vi "Handshake.vi"(5 "error in":T1) -> (19 "error out":T1)   [LabVIEW 2016]
doc: "If the path mode is waiting for a manual handshake, this VI will give this handshake and the path will be continued."
uses:
  Controls/Error_Out.ctl
  Files_ASC500/DLL/ASC500_RemoteControlV27.dll
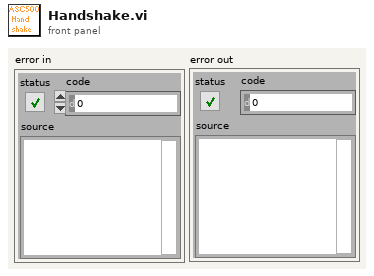
[diagram p1: front panel]
types:
  T1 = typedef "Error_Out.ctl" = errorcluster
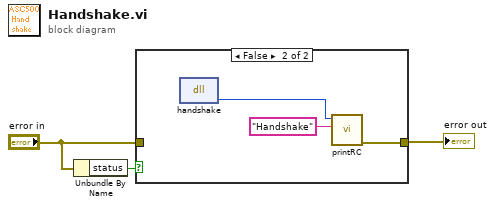
[diagram p0: block diagram]
diagram:
  n1 = Unbundle By Name("error in") -> ("status"=w3:bool)
  n2 = case shown="False" w3 {
    tunnel: [w4 w7] -> w2
    tunnel: "error in" -> [w4 _]
    frame True {
    }
    frame False {
      n3 = dll-call lib="G:/SCMOperations/Share/ELE/Produkt Information/ASC500/04 Remote Control/02 development versions/2018Nov06/Files_ASC500/DLL/ASC500_RemoteControlV27.dll" fn="handshake"() -> ("return type"=w6:i32)  [unwired: 3 in, 2 out]
      n4 = call "printRC.vi"("additional information"="Handshake", "RC"=w6) -> ("error out"=w7:T1)  [unwired: 9 in]
    }
  }
  "error out" <- w2
